vi "线性拟合.vi"() -> ()   [LabVIEW 2018]
uses:
  <vilib>/Analysis/6fits.llb/Curve Fitting Criteria.ctl
  <vilib>/Analysis/NI_AALPro.lvlib
panel:
  in  "停止":bool
  out "residue":dbl caption="残差"
  out "intercept":dbl caption="截距"
  out "slope":dbl caption="斜率"
  in  "tolerance":dbl=0.0001 caption="容差" format="%#_3g"
  in  "method":T1 caption="方法" items=["最小二乘", "最小绝对残差", "Bisquare"]
  in  "Weight":dbl[](array[numeric]) caption="权重"
  in  "数组 2":dbl[](array[numeric])
  in  "数组":dbl[](array[numeric])
  out "拟合后":dbl[](graph)
  out "波形图 2":dbl[](graph)
  out "波形图":dbl[](graph)
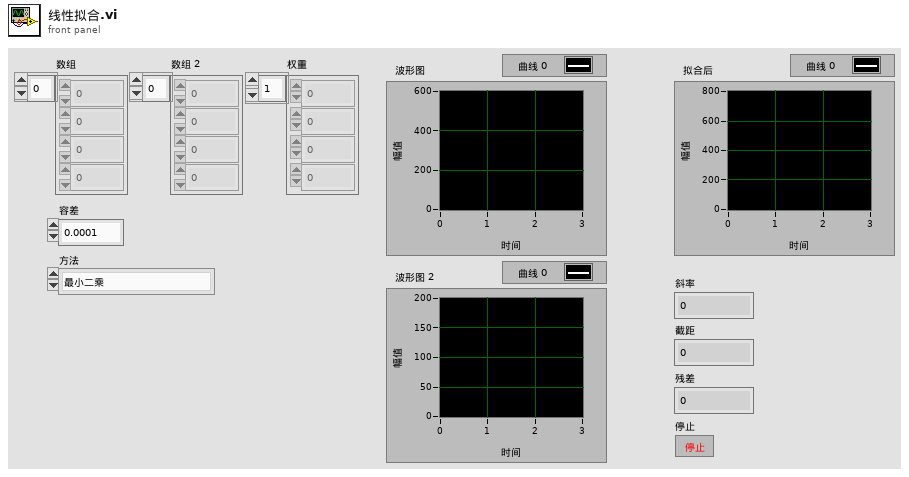
[diagram p1: front panel]
types:
  T1 = typedef "NI_AALPro.lvlib/Curve Fitting Criteria.ctl" = u16
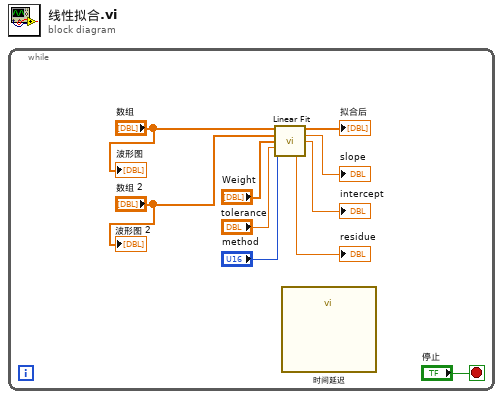
[diagram p0: block diagram]
diagram:
  n1 = while {
    stop <- "停止" stop-if-true
    n2 = call <vilib>:"Linear Fit.vi"("Y"="数组", "X"="数组 2", "Weight"="Weight", "tolerance"="tolerance", "method"="method") -> ("Best Linear Fit"=→"拟合后":dbl[], "slope"=→"slope":dbl, "intercept"=→"intercept":dbl, "residue"=→"residue":dbl)  [unwired: 6 in, 1 out]
    n3 = call "时间延迟"() -> ()  [unwired: 11 in, 1 out]
    "波形图" <- "数组"
    "波形图 2" <- "数组 2"
  }
